vi "Scan for Motors.vi"(7 "Search Timeout (10000 ms)":u32=10000, 8 "error in (no error)":errorcluster, 9 "Ending ID (253)":u8=253, 10 "Starting ID (0)":u8, 11 "Dynamixel Motor in":refnum<class "Dynamixel Motor.lvclass">) -> (0 "error out":errorcluster, 2 "Motors IDs Found":u8[](array[numeric]), 3 "Dynamixel Motor out":refnum<class "Dynamixel Motor.lvclass">)   [LabVIEW 2016, in "Dynamixel Motor.lvclass"]
doc: "Scans sequentially for motors between <b>Starting ID</b> and <b>Ending ID</b> for no longer than <b>Search Timeout</b>. If all of the motors do not have unique IDs, then motors with duplicate IDs may not be found."
uses:
  <instrlib>/Dynamixel Motor/HAIOL/Dynamixel Motor.lvclass
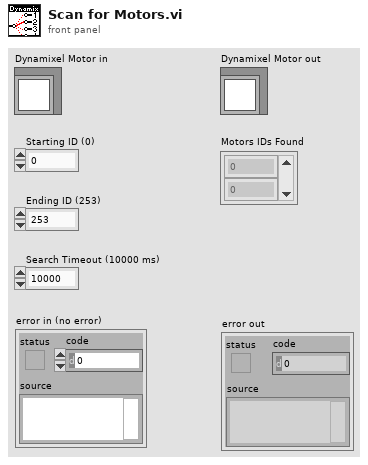
[diagram p1: front panel]
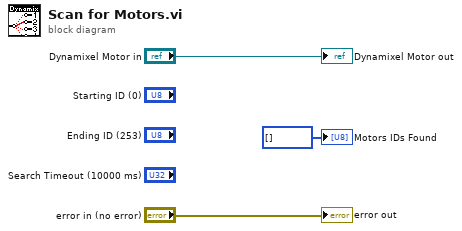
[diagram p0: block diagram]
diagram:
  "error out" <- "error in (no error)"
  "Dynamixel Motor out" <- "Dynamixel Motor in"
  "Motors IDs Found" <- u8[] [] ("Motors IDs Found")
